vi "Initalize.vi"(8 "error in (no error)":errorcluster, 9 "Section":string, 10 "Config Path":path, 11 "MAS in":refnum<class "MAS.lvclass">) -> (0 "error out":errorcluster, 3 "MAS out":refnum<class "MAS.lvclass">)   [LabVIEW 2022 SP3, in "MAS.lvclass"]
uses:
  MAS.lvclass
  C:/Users/Josh.Thibeault/Desktop/MAS/Base/Base.lvclass
  Settings.ctl
  Base/Base.lvclass/Base.ctl
  MAS.lvclass/MAS.ctl
  b142521d-98f7-4923-9666-3793bf2d8571.vi
  Base/Accessors/Write Config Path.vi
  Base/Accessors/Write Section.vi
  <vilib>/Utility/LVClass/Get LV Class Default Value.vi
  iMotion Controller/iMotion Controller.lvclass
  Read Configs/Read Configs Sections.lvlib
panel:
  out "Settings":T1
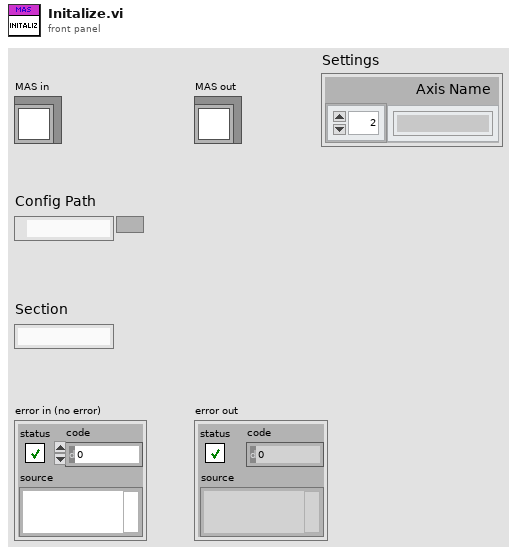
[diagram p1: front panel]
types:
  T1 = typedef "MAS.lvclass/Settings.ctl" = cluster{"Axis Name":string[]}
  T2 = typedef "Read Configs Sections.lvlib/Section Data.ctl" = cluster{"Componets":string[], "Path":path, "Section":string}
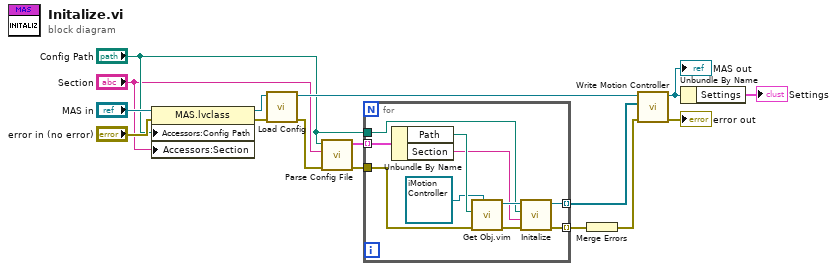
[diagram p0: block diagram]
diagram:
  n1 = property class="MAS.lvclass"(reference="MAS in", error in="error in (no error)", "Accessors:Config Path"="Config Path", "Accessors:Section"="Section") -> (reference out=w3:refnum<class "MAS.lvclass">, error out=w7:errorcluster)
  n2 = call-dynamic "Load Config.vi"("error in (no error)"=w7, "MAS in"=w3) -> ("error out"=w8:errorcluster, "MAS out"=w10:refnum<class "MAS.lvclass">)  [unwired: 8 in]
  n3 = call "Parse Config File.vi"("error in (no error)"=w8, "Section"="Section", "Config Path"="Config Path") -> ("error out"=w14:errorcluster, "Array"=w16:T2[])  [unwired: 7 in]
  n4 = for {
    tunnel: w16 -> [w26] mode=indexing
    tunnel: "Config Path" -> [w22]
    tunnel: [w17] -> w15 mode=indexing
    tunnel: w14 -> [w20]
    tunnel: [w18] -> w13 mode=indexing
    n5 = Unbundle By Name(w26) -> ("Path"=w25:path, "Section"=w21:string)
    n6 = call "Get Obj.vim"("LabVIEW Object 2"=refnum<class "iMotion Controller.lvclass"> refnum ("iMotion Controller.lvclass"), "error in (no error)"=w20, "Path"=w25) -> ("error out"=w19:errorcluster, "LabVIEW Object"=w23:refnum<class "iMotion Controller.lvclass">)  [unwired: 7 in]
    n7 = call-dynamic "Initalize.vi"("error in (no error)"=w19, "Section"=w21, "Config Path"=w22, "Dynamic Load in"=w23) -> ("error out"=w18:errorcluster, "Dynamic Load out"=w17:refnum<class "iMotion Controller.lvclass">)  [unwired: 6 in]
  }
  n8 = Merge Errors(w13) -> (w12:errorcluster)
  n9 = call "Write Motion Controller .vi"("error in (no error)"=w12, "Motion Controller"=w15, "MAS in"=w10) -> ("error out"=→"error out":errorcluster, "MAS out"=w2:refnum<class "MAS.lvclass">)  [unwired: 7 in]
  "MAS out" <- w2
  n10 = Unbundle By Name(w2) -> ("Settings"=→"Settings":T1)
